vi "GF_UpdateGraphData.vi"(1 "error in (no error)":errorcluster, 2 "Wavenames Array":string[](array[string]), 3 "Waveform Array":waveform(dbl)[](array[waveform]), 4 "Graph Ref Array":refnum<vi>[](array[refnum])) -> (0 "error out":errorcluster)   [LabVIEW 2016]
panel:
  in  "Select Channels":i32[](listbox)=[128, 129, 130]
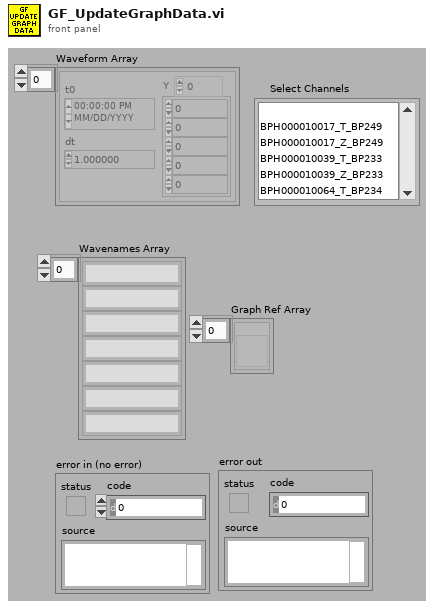
[diagram p1: front panel]
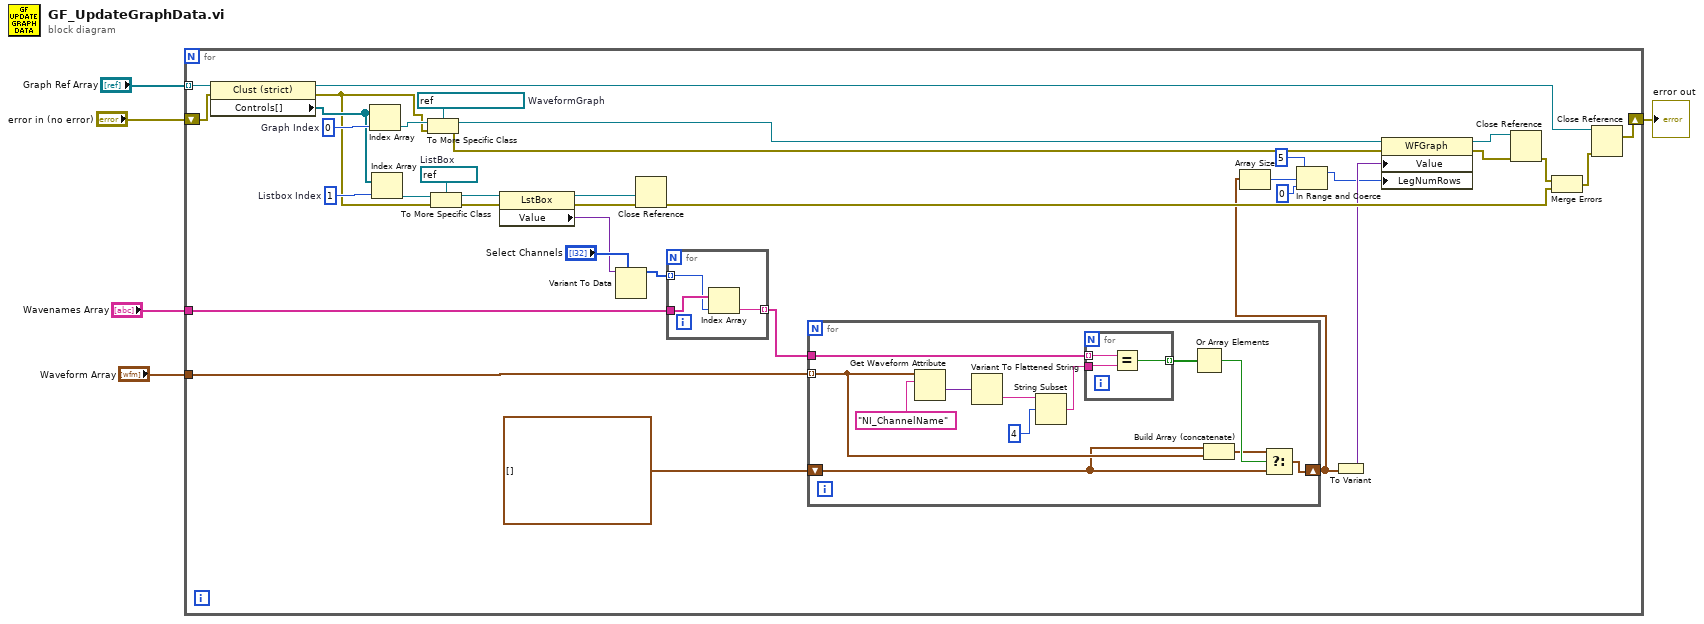
[diagram p0: block diagram]
diagram:
  n1 = for {
    tunnel: "Graph Ref Array" -> [w33] mode=indexing
    tunnel: "Wavenames Array" -> [w18]
    tunnel: "Waveform Array" -> [w16]
    shift-right: [w12] -> w5
    shift-left: "error in (no error)" -> [w11]
    w30 = refnum<vi> refnum  # ListBox
    w32 = 1  # Listbox Index
    w39 = refnum<vi> refnum  # WaveformGraph
    w41 = 0  # Graph Index
    n2 = property class="Clust (strict)"(reference=w33, error in=w11) -> (reference out=w34:refnum<vi>, error out=w21:errorcluster, "Controls[]"=w31:refnum<vi>[])
    n3 = Index Array(array=w31, index=w41) -> (element=w40:refnum<vi>)
    n4 = Index Array(array=w31, index=w32) -> (element=w29:refnum<vi>)
    n5 = To More Specific Class(target class=w39, reference=w40, error in=w21) -> (specific class reference=w38:refnum<vi>, error out=w35:errorcluster)
    n6 = To More Specific Class(target class=w30, reference=w29, error in=w21) -> (specific class reference=w28:refnum<vi>, error out=w22:errorcluster)
    n7 = property class="LstBox"(reference=w28, error in=w22) -> (reference out=w27:refnum<vi>, error out=w23:errorcluster, "Value"=w19:variant)
    n8 = Variant To Data(type="Select Channels", Variant=w19) -> (data=w17:i32[])  [unwired: 1 in, 1 out]
    n9 = Close Reference(reference=w27, error in (no error)=w23) -> (error out=w26:errorcluster)
    n10 = for {
      tunnel: w18 -> [w59]
      tunnel: w17 -> [w58] mode=indexing
      tunnel: [w57] -> w15 mode=indexing
      n11 = Index Array(array=w59, index=w58) -> (element=w57:string)
    }
    n12 = for {
      tunnel: w16 -> [w47] mode=indexing
      tunnel: w15 -> [w49]
      shift-right: [w44] -> w10
      shift-left: waveform(dbl)[] [] -> [w42]
      n13 = Get Waveform Attribute(6:"NI_ChannelName", 7:w47) -> (1:w52:variant)  [unwired: 2 in, 3 out]
      n14 = Variant To Flattened String(Variant=w52) -> (data string=w51:string)  [unwired: 1 out]
      n15 = String Subset(string=w51, offset (0)=4) -> (substring=w48:string)  [unwired: 1 in]
      n16 = for {
        tunnel: w49 -> [w56] mode=indexing
        tunnel: w48 -> [w55]
        tunnel: [w54] -> w46 mode=indexing
        n17 = Equal?(x=w56, y=w55) -> (x = y?=w54:bool)
      }
      n18 = Or Array Elements(Boolean array=w46) -> (logical OR=w45:bool)
      n19 = Build Array (concatenate)(w42, w47) -> (w43:waveform(dbl)[])
      n20 = Select(t=w43, s=w45, f=w42) -> (s? t:f=w44:waveform(dbl)[])
    }
    n21 = Array Size(array=w10) -> (size(s)=w9:i32)
    n22 = In Range and Coerce(upper limit=5, x=w9, lower limit=0) -> (coerced(x)=w8:i32)  [unwired: 1 out]
    n23 = To Variant(anything=w10) -> (Variant=w13:variant)
    n24 = property class="WFGraph"(reference=w38, error in=w35, "Value"=w13, "LegNumRows"=w8) -> (reference out=w37:refnum<vi>, error out=w36:errorcluster)
    n25 = Close Reference(reference=w37, error in (no error)=w36) -> (error out=w25:errorcluster)
    n26 = Merge Errors(w25, w26) -> (w24:errorcluster)
    n27 = Close Reference(reference=w34, error in (no error)=w24) -> (error out=w12:errorcluster)
  }
  "error out" <- w5
